vi "Add Shortcut Menu Items.vi"(9 "Container State":T3, 10 "Display State In":T1 caption="State", 11 "Menu in":refnum<k9>) -> ()   [LabVIEW 2011, in "Taskbar Progress Bar.xctl"]
uses:
  Taskbar Progress Bar.xctl
  <vilib>/_xctls/Container State.ctl
  Abilities/PB State.ctl
  TypeDefs/Dispaly State Change Methods.ctl
  <vilib>/_xctls/XControlSupport.lvlib
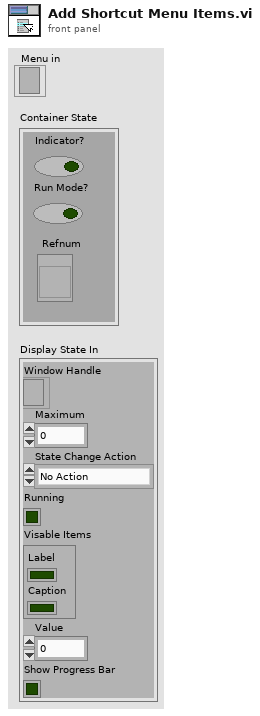
[diagram p1: front panel]
types:
  T1 = typedef "Taskbar Progress Bar.xctl/PB State.ctl" = cluster{"Window Handle":refnum<k24>, "Maximum":u64, "State Change Action":T2, "Running":bool, "Visable Items":cluster{"Label":bool, "Caption":bool}, "Value":u64, "Show Progress Bar":bool}
  T2 = typedef "Taskbar Progress Bar.xctl/Dispaly State Change Methods.ctl" = enum16{"No Action", "Created", "Method - Initialize", "Method - Increment", "Method - Pause", "Method - Error", "Method - Finish", "Property - Show Progress Bar"}
  T3 = typedef "XControlSupport.lvlib/Container State.ctl" = cluster{"Indicator?":bool, "Run Mode?":bool, " Refnum":refnum<vi>}
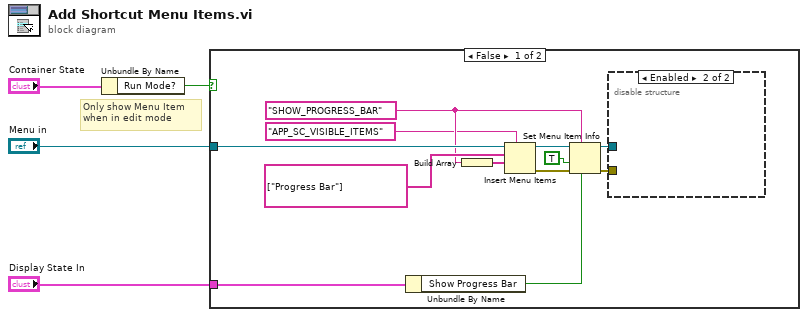
[diagram p0: block diagram]
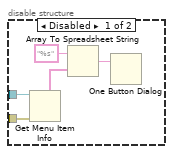
[diagram p2: hidden frame]
diagram:
  # "Only show Menu Item\nwhen in edit mode"
  n1 = Unbundle By Name("Container State") -> ("Run Mode?"=w1:bool)
  n2 = case shown="False" w1 {
    tunnel: "Menu in" -> [w16 _]
    tunnel: "Display State In" -> [w13 _]
    frame False {
      w9 = "SHOW_PROGRESS_BAR"
      n3 = Unbundle By Name(w13) -> ("Show Progress Bar"=w12:bool)
      n4 = Build Array(w9) -> (w8:string[])
      n5 = Insert Menu Items(5:"APP_SC_VISIBLE_ITEMS" ("menu tag"), 7:w8, 8:string[] ["Progress Bar"] ("item names"), 9:w16) -> (0:w14:errorcluster, 3:w15:refnum<k9>)  [unwired: 2 in, 1 out]
      n6 = Set Menu Item Info(6:w12, 7:w9, 8:w14, 9:TRUE ("enabled"), 11:w15) -> (0:w6:errorcluster, 3:w7:refnum<k9>)  [unwired: 2 in]
      n7 = disable-structure shown="Enabled" {
        disable-tunnel: w7 -> [w21 _]
        disable-tunnel: w6 -> [w20 _]
        frame Disabled {
          n8 = Get Menu Item Info(8:w20, 11:w21) -> (5:w19:string[])  [unwired: 1 in, 6 out]
          n9 = Array To Spreadsheet String(array=w19, 3:"%s" ("format string")) -> (spreadsheet string=w17:string)  [unwired: 1 in]
          n10 = One Button Dialog(message=w17) -> ()  [unwired: 1 in, 1 out]
        }
        frame Enabled {
        }
      }
    }
    frame True {
    }
  }
